vi "Material-Application-Dir-User.vi"(11 "error in":errorcluster) -> (4 "Deploy User App Data Directory":path, 15 "error out":errorcluster)   [LabVIEW 2013]
uses:
  Material-Application-DeploymentConstants.vi
panel:
  # "Inputs"
  # "Outputs"
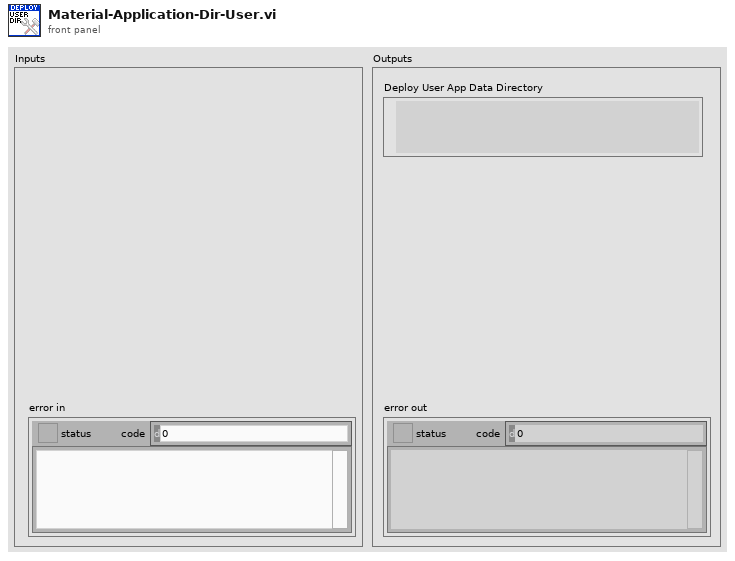
[diagram p1: front panel]
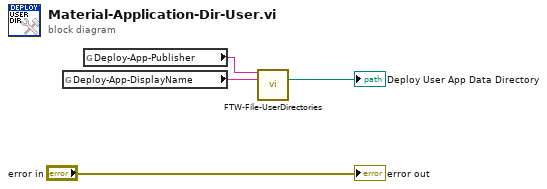
[diagram p0: block diagram]
diagram:
  n1 = global read "Material-Application-DeploymentConstants.vi" "Deploy-App-DisplayName"() -> (w1:string)
  n2 = global read "Material-Application-DeploymentConstants.vi" "Deploy-App-Publisher"() -> (w2:string)
  n3 = call "FTW-File-UserDirectories.vi"("Publisher (Organization)"=w2, "Application (Product Name)"=w1) -> ("User Application Data Dir"=→"Deploy User App Data Directory":path)  [unwired: 10 in, 3 out]
  "error out" <- "error in"
